vi "SanitizeScriptStringArray.vi"(11 "Array in":string[](array[string])) -> (3 "Array out":string[](array[string]))   [LabVIEW 2018, in "Test.lvclass"]
uses:
  Test.lvclass
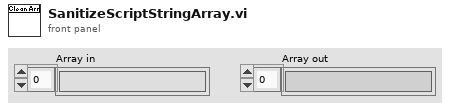
[diagram p1: front panel]
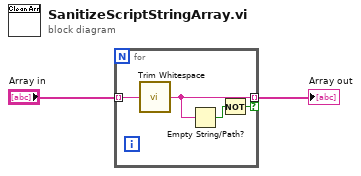
[diagram p0: block diagram]
diagram:
  n1 = for {
    tunnel: "Array in" -> [w6] mode=indexing
    tunnel: [w5] -> w2 mode=indexing if=w3
    n2 = call <vilib>:"Trim Whitespace.vi"("string"=w6) -> ("trimmed string"=w5:string)  [unwired: 1 in]
    n3 = Empty String/Path?(string/path=w5) -> (empty?=w4:bool)
    n4 = Not(x=w4) -> (.not. x?=w3:bool)
  }
  "Array out" <- w2
